vi "GCD of P(x) and Q(x) (CDB).vi"(8 "algorithm":u16(ring) items=["Euclidean", "Approximate GCD"], 9 "tolerance":dbl=1e-08, 10 "Q(x)":cdb[](array[numeric]) format="%#.6g", 11 "P(x)":cdb[](array[numeric]) format="%#.6g") -> (0 "error":i32, 3 "Greatest Common Divisor":cdb[](array[numeric]) format="%#.6g")   [LabVIEW 2018, in "NI_AALPro.lvlib"]
doc: "Computes the greatest common divisor for two polynomials <B>P(x)</B> and <B>Q(x)</B> with the <B>tolerance</B> you specify. The data types you wire to the <B>P(x)</B> and <B>Q(x)</B> inputs determine the polymorphic instance to use."
uses:
  <vilib>/Analysis/NI_AALPro.lvlib
  RMS (DBL).vi
  Polynomial GCD Pair (CDB).vi
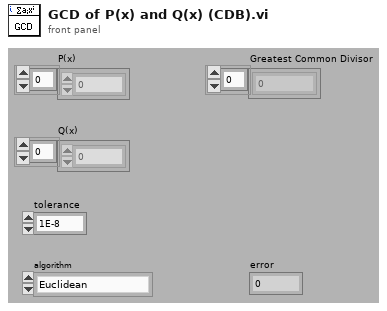
[diagram p1: front panel]
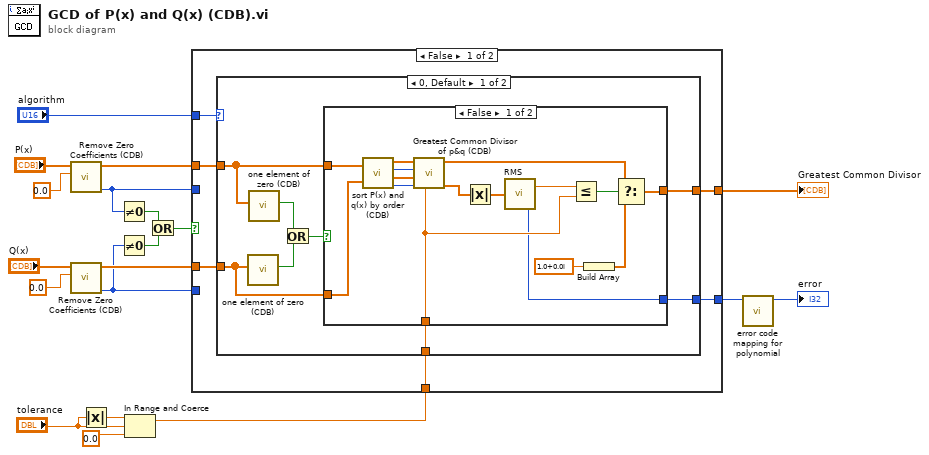
[diagram p0: block diagram]
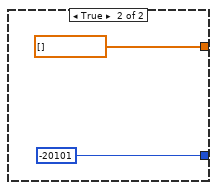
[diagram p2: hidden frame]
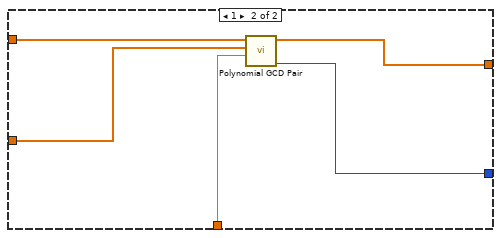
[diagram p3: hidden frame]
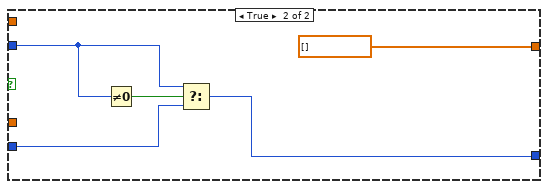
[diagram p4: hidden frame]
diagram:
  n1 = call "Remove Zero Coefficients (CDB).vi"("threshold"=0.0, "P(x) In"="P(x)") -> ("error"=w6:i32, "P(x) Out"=w16:cdb[])  [unwired: 7 in, 1 out]
  n2 = call "Remove Zero Coefficients (CDB).vi"("threshold"=0.0, "P(x) In"="Q(x)") -> ("error"=w5:i32, "P(x) Out"=w15:cdb[])  [unwired: 7 in, 1 out]
  n3 = Absolute Value(x="tolerance") -> (abs(x)=w12:dbl)
  n4 = Not Equal To 0?(x=w6) -> (x != 0?=w4:bool)
  n5 = Not Equal To 0?(x=w5) -> (x != 0?=w3:bool)
  n6 = In Range and Coerce(upper limit=w12, x="tolerance", lower limit=0.0) -> (coerced(x)=w9:dbl)  [unwired: 1 out]
  n7 = Or(x=w4, y=w3) -> (x .or. y?=w2:bool)
  n8 = case shown="False" w2 {
    tunnel: [w25 cdb[] [] ("CDB")] -> w19
    tunnel: w16 -> [w24 _]
    tunnel: w15 -> [w23 _]
    tunnel: [w22 w57] -> w8
    tunnel: w9 -> [w21 _]
    tunnel: w6 -> [_ w59]
    tunnel: w5 -> [_ w58]
    tunnel: "algorithm" -> [w20 _]
    frame False {
      n9 = case shown="0, Default" w20 {
        tunnel: [w33 w53] -> w25
        tunnel: w24 -> [w31 w56]
        tunnel: w23 -> [w28 w55]
        tunnel: [w27 w52] -> w22
        tunnel: w21 -> [w26 w54]
        frame 0, Default {
          n10 = call "one element of zero (CDB).vi"("Array in"=w28) -> ("equal [0]?"=w29:bool)  [unwired: 10 in]
          n11 = call "one element of zero (CDB).vi"("Array in"=w31) -> ("equal [0]?"=w30:bool)  [unwired: 10 in]
          n12 = Or(x=w30, y=w29) -> (x .or. y?=w32:bool)
          n13 = case shown="False" w32 {
            tunnel: w31 -> [w49 _]
            tunnel: w28 -> [w48 _]
            tunnel: [w46 cdb[] []] -> w33
            tunnel: [w34 -20101 ("coef. of poly are all zero")] -> w27
            tunnel: w26 -> [w35 _]
            frame False {
              n14 = call "sort P(x) and q(x) by order (CDB).vi"("p"=w49, "q"=w48) -> ("high order polynomial"=w45:cdb[], "high order"=w44:i32, "low order polynomial"=w43:cdb[], "low order"=w42:i32)
              n15 = call "Greatest Common Divisor of p&q (CDB).vi"("tolerance"=w35, "order of q"=w42, "q"=w43, "order of p"=w44, "p"=w45) -> ("rest"=w38:cdb[], "greatest common factor"=w41:cdb[])  [unwired: 4 in, 1 out]
              n16 = Absolute Value(x=w38) -> (abs(x)=w37:dbl[])
              n17 = call-poly "RMS.vi"("X"=w37) -> ("rms value"=w36:dbl, "error"=w34:i32)
              n18 = Less Or Equal?(x=w36, y=w35) -> (x <= y?=w47:bool)
              n19 = Build Array(cdb 1.0+0.0i) -> (w39:cdb[])
              n20 = Select(t=w41, s=w47, f=w39) -> (s? t:f=w46:cdb[])
            }
            frame True {
            }
          }
        }
        frame 1 {
          n21 = call-poly "Polynomial GCD Pair.vi"("tolerance"=w54, "Q(x)"=w55, "P(x)"=w56) -> ("error"=w52:i32, "Greatest Common Divisor"=w53:cdb[])  [unwired: 5 in, 2 out]
        }
      }
    }
    frame True {
      n22 = Not Equal To 0?(x=w59) -> (x != 0?=w60:bool)
      n23 = Select(t=w59, s=w60, f=w58) -> (s? t:f=w57:i32)
    }
  }
  "Greatest Common Divisor" <- w19
  n24 = call "error code mapping for polynomial.vi"("error in"=w8) -> ("error out"=→"error":i32)  [unwired: 10 in]
